vi "Self-Test.vi"(8 "error in":errorcluster caption="error in (no error)", 11 "Resource":string) -> (0 "error out":errorcluster, 3 "Result":string)   [LabVIEW 2020, in "NI SysCfg.lvlib"]
uses:
  NI SysCfg.lvlib
  <vilib>/nisyscfg/Close (Hardware).vi
  <vilib>/nisyscfg/Close (System).vi
  <vilib>/nisyscfg/nisyscfg.lvlib
  <resource>/objmgr/niMIDebugSession.rc
  <resource>/objmgr/nicontrollersysapi.rc
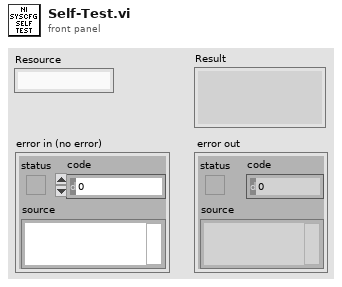
[diagram p1: front panel]
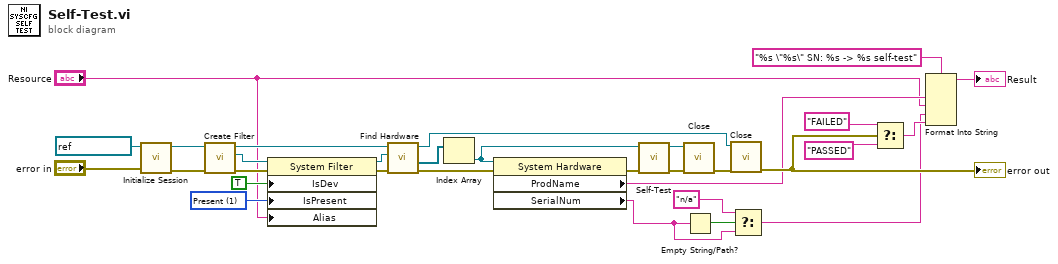
[diagram p0: block diagram]
diagram:
  w25 = 1 items=["Initializing"=-2, "Unknown"=-1, "Not Present"=0, "Present"=1] ("Devices & Chassis:Is Present")
  n1 = call <vilib>:"Initialize Session.vi"("error in (no error)"="error in", "Target (localhost)"=refnum<k21> "localhost") -> ("error out"=w24:errorcluster, "Session out"=w23:refnum<k21>)  [unwired: 8 in]
  n2 = call <vilib>:"Create Filter.vi"("error in (no error)"=w24, "Session in"=w23) -> ("error out"=w11:errorcluster, "Filter out"=w12:refnum<k20>, "Session out"=w15:refnum<k21>)  [unwired: 7 in]
  n3 = property class="System Filter"(reference=w12, error in=w11, "IsDev"=TRUE ("Is Device"), "IsPresent"=w25, "Alias"="Resource") -> (reference out=w14:refnum<k20>, error out=w13:errorcluster)
  n4 = call <vilib>:"Find Hardware.vi"("error in (no error)"=w13, "Filter in"=w14, "Session in"=w15) -> ("error out"=w7:errorcluster, "Resources out"=w18:refnum<k20>[], "Session out"=w17:refnum<k21>)  [unwired: 5 in, 1 out]
  n5 = Index Array(array=w18) -> (element=w22:refnum<k20>)  [unwired: 1 in]
  n6 = property class="System Hardware"(reference=w22, error in=w7) -> (error out=w8:errorcluster, "ProdName"=w27:string, "SerialNum"=w3:string)  [unwired: 1 out]
  n7 = call <vilib>:"Self-Test.vi"("error in (no error)"=w8, "Resource in"=w22) -> ("error out"=w19:errorcluster, "Resource out"=w21:refnum<k20>)  [unwired: 7 in, 1 out]
  n8 = call-poly <vilib>:"Close.vi"("error in (no error)"=w19, "Resource in"=w21) -> ("error out"=w20:errorcluster)  [unwired: 9 in]
  n9 = Empty String/Path?(string/path=w3) -> (empty?=w4:bool)
  n10 = call-poly <vilib>:"Close.vi"("error in (no error)"=w20, "Session in"=w17) -> ("error out"=w29:errorcluster)  [unwired: 9 in]
  "error out" <- w29
  n11 = Select(t="n/a", s=w4, f=w3) -> (s? t:f=w1:string)
  n12 = Select(t="FAILED" ("format string"), s=w29, f="PASSED" ("format string")) -> (s? t:f=w5:string)
  n13 = Format Into String(format string="%s \"%s\" SN: %s -> %s self-test", w27, "Resource", w1, w5) -> (resulting string=→"Result":string)  [unwired: 2 in, 1 out]
